vi "DL950RMS.vi"() -> ()   [LabVIEW 2019]
uses:
  <instrlib>/Yokogawa DL950 Series/Yokogawa DL950 Series.lvlib
panel:
  out "error out 2":errorcluster
  in  "Time Division (12: 1ms)":i32(ring)=19 items=["100ns", "200ns", "500ns", "1us", "2us", "5us", "10us", "20us", "50us", "100us", "200us", "500us", "1ms", "2ms", "5ms", "10ms", "20ms", "50ms", "100ms", "200ms", "500ms", "1s", "2s", "3s", "4s", "5s", "6s", "10s", "20s", "30s", "1min", "2min", "3min", "4min", "5min", "6min", "10min", "12min", "30min", "1hour", "2hour", "3hour", "4hour", "5hour", "6hour", "8hour", "10hour", "12hour", "1day", "2day", "3day", "4day", "5day"]
  in  "Acquisition Mode (0: Normal)":i32(ring) items=["Normal", "Average", "Envelope"]
  in  "Record Length (0: 10k)":i32(ring) items=["10k", "25k", "50k", "100k", "250k", "500k", "1M", "2.5M", "5M", "10M", "25M", "50M", "100M", "250M", "500M", "1G", "2G", "4G", "5G", "10G", "20G", "50G"]
  out "error out":errorcluster
  out "Array":dbl[](array[numeric])
  in  "items":i32[](array[ring]) items=["Peak to Peak", "Amplitude", "Max", "Min", "High", "Low", "Average", "Middle", "Rms", "Standard Deviation", "+Overshoot", "-Overshoot", "Rise", "Fall", "Frequency", "Period", "+Width", "-Width", "Duty Cycle", "Pulse Count", "Burst1 Width", "Burst2 Width", "Average Frequency", "Average Period", "Int1TY", "Int2TY"]
  in  "enable":bool[](array[boolean])
  in  "Source (1: CH1)":u16(ring)=1 items=["", "CH1", "CH2", "CH3", "CH4", "CH5", "CH6", "CH7", "CH8", "CH9", "CH10", "CH11", "CH12", "CH13", "CH14", "CH15", "CH16", "MATH1", "MATH2", "MATH3", "MATH4", "MATH5", "MATH6", "MATH7", "MATH8", "EVENT"]
  in  "Sub Channel (0: None)":i16(ring) items=["None", "SCH1", "SCH2", "SCH3", "SCH4", "SCH5", "SCH6", "SCH7", "SCH8", "SCH9", "SCH10", "SCH11", "SCH12", "SCH13", "SCH14", "SCH15", "SCH16", "SCH17", "SCH18", "SCH19", "SCH20", "SCH21", "SCH22", "SCH23", "SCH24", "SCH25", "SCH26", "SCH27", "SCH28", "SCH29", "SCH30", "SCH31", "SCH32", "SCH33", "SCH34", "SCH35", "SCH36", "SCH37", "SCH38", "SCH39", "SCH40", "SCH41", "SCH42", "SCH43", "SCH44", "SCH45", "SCH46", "SCH47", "SCH48", "SCH49", "SCH50", "SCH51", "SCH52", "SCH53", "SCH54", "SCH55", "SCH56", "SCH57", "SCH58", "SCH59", "SCH60", "SCH61", "SCH62", "SCH63", "SCH64"]
  in  "Timeout (10000 ms)":u32=10000
  out "Name of Items":string[](array[string])
  in  "Vertical Division (20: 50)":i32(ring)=20 items=["0.1m", "0.2m", "0.5m", "1m", "2m", "5m", "10m", "20m", "50m", "100m", "200m", "500m", "1", "2", "4", "5", "8", "10", "20", "40", "50", "80", "100", "200", "400", "500", "800", "1k", "2k", "4k", "5k", "8k", "10k", "20k", "25k", "50k", "100k", "250k", "500k", "1000k"]
  in  "Vertical Coupling (1: DC)":i32(ring)=1 items=["AC", "DC", "Ground", "AC-RMS", "DC-RMS"]
  in  "VISA resource name":refnum<visa-resource-name>="TCPIP0::192.168.0.100::inst0::INSTR"
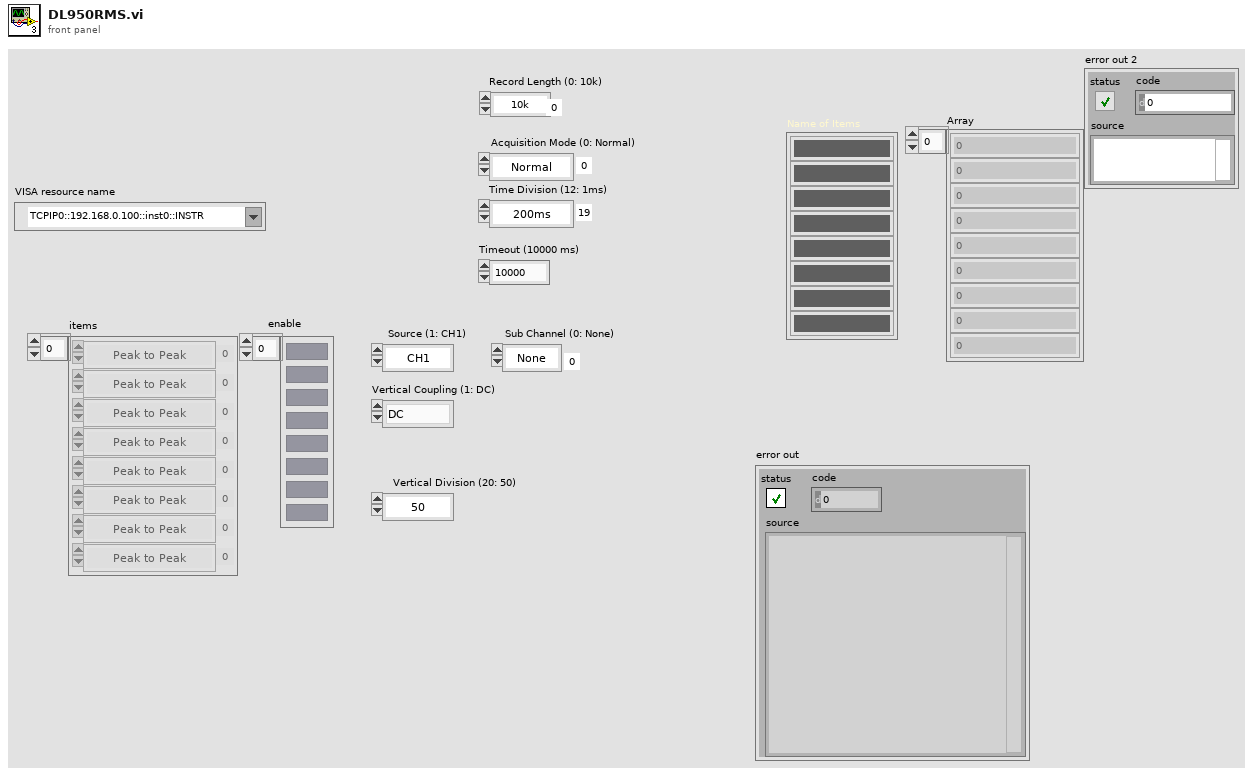
[diagram p1: front panel]
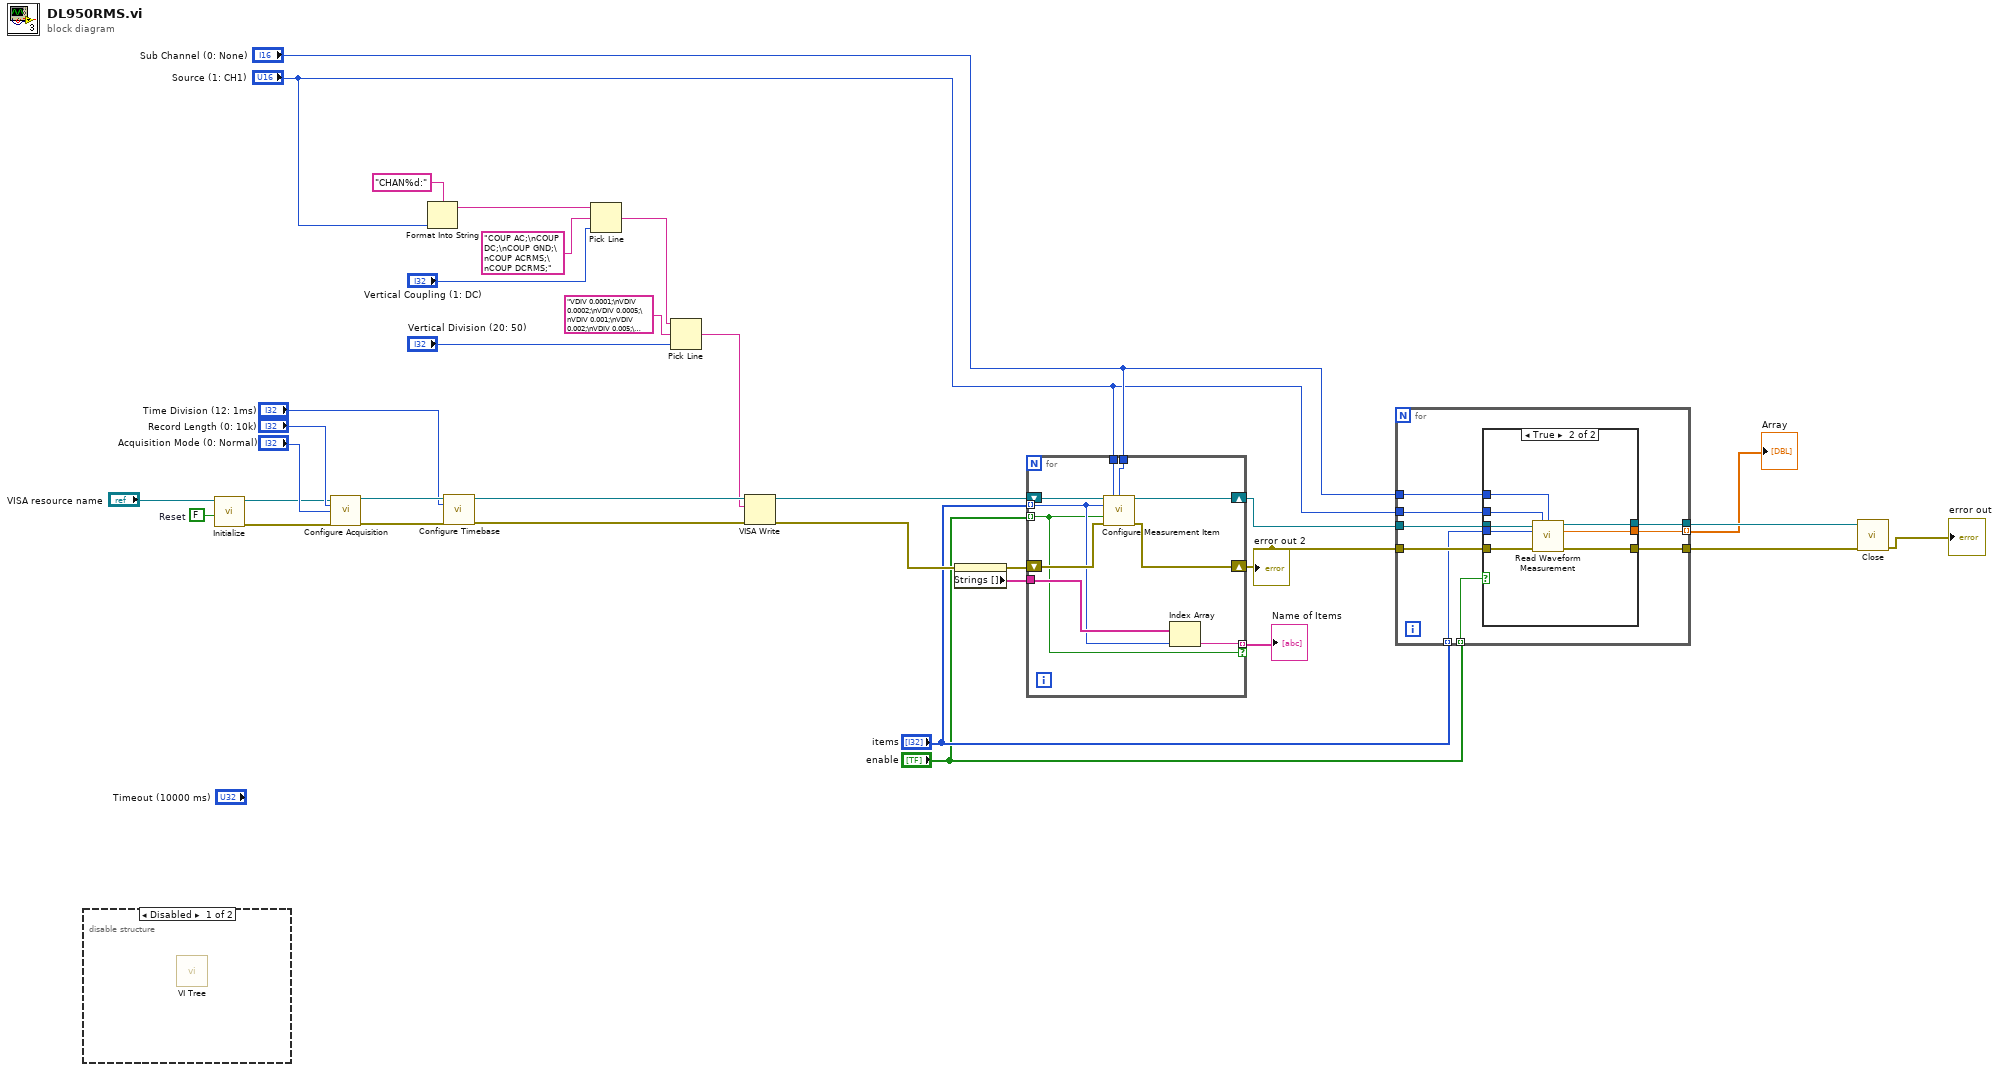
[diagram p0: block diagram]
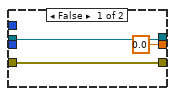
[diagram p2: hidden frame]
diagram:
  w34 = FALSE  # Reset
  n1 = disable-structure shown="Disabled" {
    frame Disabled {
      n2 = call <instrlib>:"VI Tree.vi"() -> ()  [unwired: 12 in]
    }
    frame Enabled {
    }
  }
  n3 = call <instrlib>:"Initialize.vi"("Reset (True)"=w34, "VISA resource name"="VISA resource name") -> ("error out"=w24:errorcluster, "VISA resource name out"=w25:refnum<visa-resource-name>)  [unwired: 8 in]
  n4 = call <instrlib>:"Configure Acquisition.vi"("VISA resource name"=w25, "Record Length (0: 10k)"="Record Length (0: 10k)", "Acquisition Mode (0: Normal)"="Acquisition Mode (0: Normal)", "error in (no error)"=w24) -> ("VISA resource name out"=w28:refnum<visa-resource-name>, "error out"=w27:errorcluster)  [unwired: 10 in]
  n5 = Format Into String ("文字列にフォーマット")(format string="CHAN%d:", "Source (1: CH1)") -> (resulting string=w7:string)  [unwired: 2 in, 1 out]
  n6 = call <instrlib>:"Configure Timebase.vi"("VISA resource name"=w28, "Time Division (12: 1ms)"="Time Division (12: 1ms)", "error in (no error)"=w27) -> ("VISA resource name out"=w20:refnum<visa-resource-name>, "error out"=w19:errorcluster)  [unwired: 11 in]
  n7 = Pick Line ("ライン選択")(string ("")=w7, multi-line string="COUP AC;\nCOUP DC;\nCOUP GND;\nCOUP ACRMS;\nCOUP DCRMS;", line index="Vertical Coupling (1: DC)") -> (output string=w5:string)
  n8 = Pick Line ("ライン選択")(string ("")=w5, multi-line string="VDIV 0.0001;\nVDIV 0.0002;\nVDIV 0.0005;\nVDIV 0.001;\nVDIV 0.002;\nVDIV 0.005;\nVDIV 0.01;\nVDIV 0.02;\nVDIV 0.05;\nVDIV 0.1;\nVDIV 0.2;\nVDIV 0.5;\nVDIV 1;\nVDIV 2;\nVDIV 4;\nVDIV 5;\nVDIV 8;\nVDIV 10;\nVDIV 20;\nVDIV 40;\nVDIV 50;\nVDIV 80;\nVDIV 100;\nVDIV 200;\nVDIV 400;\nVDIV 500;\nVDIV 800;\nVDIV 1000;\nVDIV 2000;\nVDIV 4000;\nVDIV 5000;\nVDIV 8000;\nVDIV 10000;\nVDIV 20000;\nVDIV 25000;\nVDIV 50000;\nVDIV 100000;\nVDIV 250000;\nVDIV 500000;\nVDIV 1000000;", line index="Vertical Division (20: 50)") -> (output string=w2:string)
  n9 = VISA Write ("VISA書き込み")(VISA resource name=w20, write buffer=w2, error in (no error)=w19) -> (VISA resource name out=w22:refnum<visa-resource-name>, error out=w21:errorcluster)  [unwired: 1 out]
  n10 = property on="Measurement Item (0: Peak to Peak)" class="Ring (strict)"(error in=w21) -> (error out=w15:errorcluster, "Strings []"=w14:string[])  [unwired: 1 in, 1 out]
  n11 = for {
    shift-right: [w43] -> w11
    shift-left: w22 -> [w44]
    shift-right: [w41] -> w12
    shift-left: w15 -> [w42]
    tunnel: "enable" -> [w37] mode=indexing
    tunnel: "items" -> [w39] mode=indexing
    tunnel: w14 -> [w40]
    tunnel: [w38] -> w13 mode=indexing if=w37
    tunnel: "Source (1: CH1)" -> [w36]
    tunnel: "Sub Channel (0: None)" -> [w35]
    n12 = call <instrlib>:"Configure Measurement Item.vi"("VISA resource name"=w44, "Source (1: CH1)"=w36, "Sub Channel (0: None)"=w35, "Measurement Item (0: Peak to Peak)"=w39, "Enable Measurement Item (False)"=w37, "error in (no error)"=w42) -> ("VISA resource name out"=w43:refnum<visa-resource-name>, "error out"=w41:errorcluster)  [unwired: 8 in]
    n13 = Index Array(array=w40, index=w39) -> (element=w38:string)
  }
  "Name of Items" <- w13
  "error out 2" <- w12
  n14 = for {
    tunnel: w11 -> [w53]
    tunnel: [w52] -> w32
    tunnel: w12 -> [w51]
    tunnel: [w50] -> w31
    tunnel: "items" -> [w49] mode=indexing
    tunnel: "enable" -> [w48] mode=indexing
    tunnel: "Source (1: CH1)" -> [w47]
    tunnel: [w46] -> w18 mode=indexing
    tunnel: "Sub Channel (0: None)" -> [w45]
    n15 = case shown="True" w48 {
      tunnel: w53 -> [w56 w64]
      tunnel: [w56 w63] -> w52
      tunnel: w51 -> [w55 w62]
      tunnel: [w55 w61] -> w50
      tunnel: w49 -> [_ w60]
      tunnel: w47 -> [_ w59]
      tunnel: [0.0 ("Measurement Value") w58] -> w46
      tunnel: w45 -> [_ w57]
      frame False {
      }
      frame True {
        n16 = call <instrlib>:"Read Waveform Measurement.vi"("VISA resource name"=w64, "Source (1: CH1)"=w59, "Sub Channel (0: None)"=w57, "Measurement Item (0: Peak to Peak)"=w60, "error in (no error)"=w62) -> ("VISA resource name out"=w63:refnum<visa-resource-name>, "Measurement Value"=w58:dbl, "error out"=w61:errorcluster)  [unwired: 8 in]
      }
    }
  }
  "Array" <- w18
  n17 = call <instrlib>:"Close.vi"("error in (no error)"=w31, "VISA resource name"=w32) -> ("error out"=→"error out":errorcluster)  [unwired: 9 in]
